vi "Write Key (U32).vi"(7 "Section Name":string, 8 "error in (no error)":errorcluster, 9 "Value":u32, 10 "Key Name":string, 11 "Config in":T1) -> (0 "error out":errorcluster, 2 "Key Replaced?":bool, 3 "Config out":T1)   [LabVIEW 2022 SP3, in "LabVIEW-Config.lvlib"]
uses:
  LabVIEW-Config.lvlib
  Config.ctl
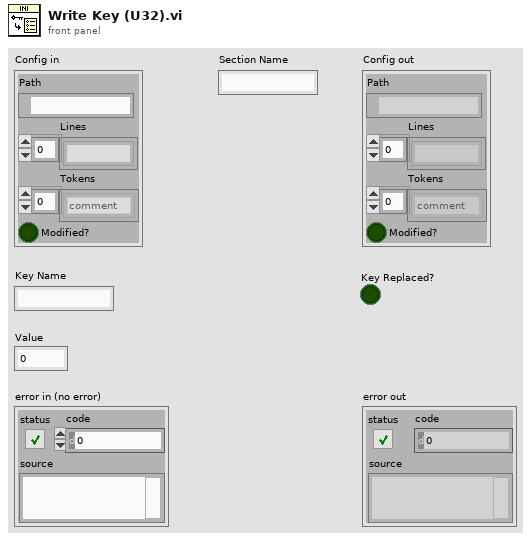
[diagram p1: front panel]
types:
  T1 = typedef "LabVIEW-Config.lvlib/Config.ctl" = cluster{"Path":path, "Lines":string[], "Tokens":enum8{"comment", "section", "key"}[], "Modified?":bool}
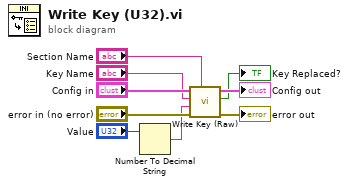
[diagram p0: block diagram]
diagram:
  n1 = Number To Decimal String(number="Value") -> (decimal integer string=w2:string)  [unwired: 1 in]
  n2 = call "Write Key (Raw).vi"("Section Name"="Section Name", "error in (no error)"="error in (no error)", "Content"=w2, "Key Name"="Key Name", "Config in"="Config in") -> ("error out"=→"error out":errorcluster, "Key Replaced?"=→"Key Replaced?":bool, "Config out"=→"Config out":T1)  [unwired: 4 in]
